vi "5.SFTP.vi"() -> ()   [LabVIEW 2012]
uses:
  UnderAutomation.UniversalRobots/UnderAutomation.UniversalRobots.lvlib
panel:
  in  "Directory to create":string
  out "Directory creation error":errorcluster
  in  "Create directory":bool
  out "Delete error":errorcluster
  in  "File or directory to delete":string
  in  "Delete":bool
  out "Download error":errorcluster
  out "Upload error":errorcluster
  out "List directory error":errorcluster
  in  "Upload":bool
  in  "Local Path":path
  in  "Robot Path":string
  in  "stop":bool
  in  "Robot Path":string
  out "DirectoryItems":T1(array[cluster])
  in  "List directory":bool
  in  "Download":bool
  out "Programs 2":string[](array[string])
  in  "Enumerate installations":bool
  in  "Enumerate programs":bool
  out "Programs":string[](array[string])
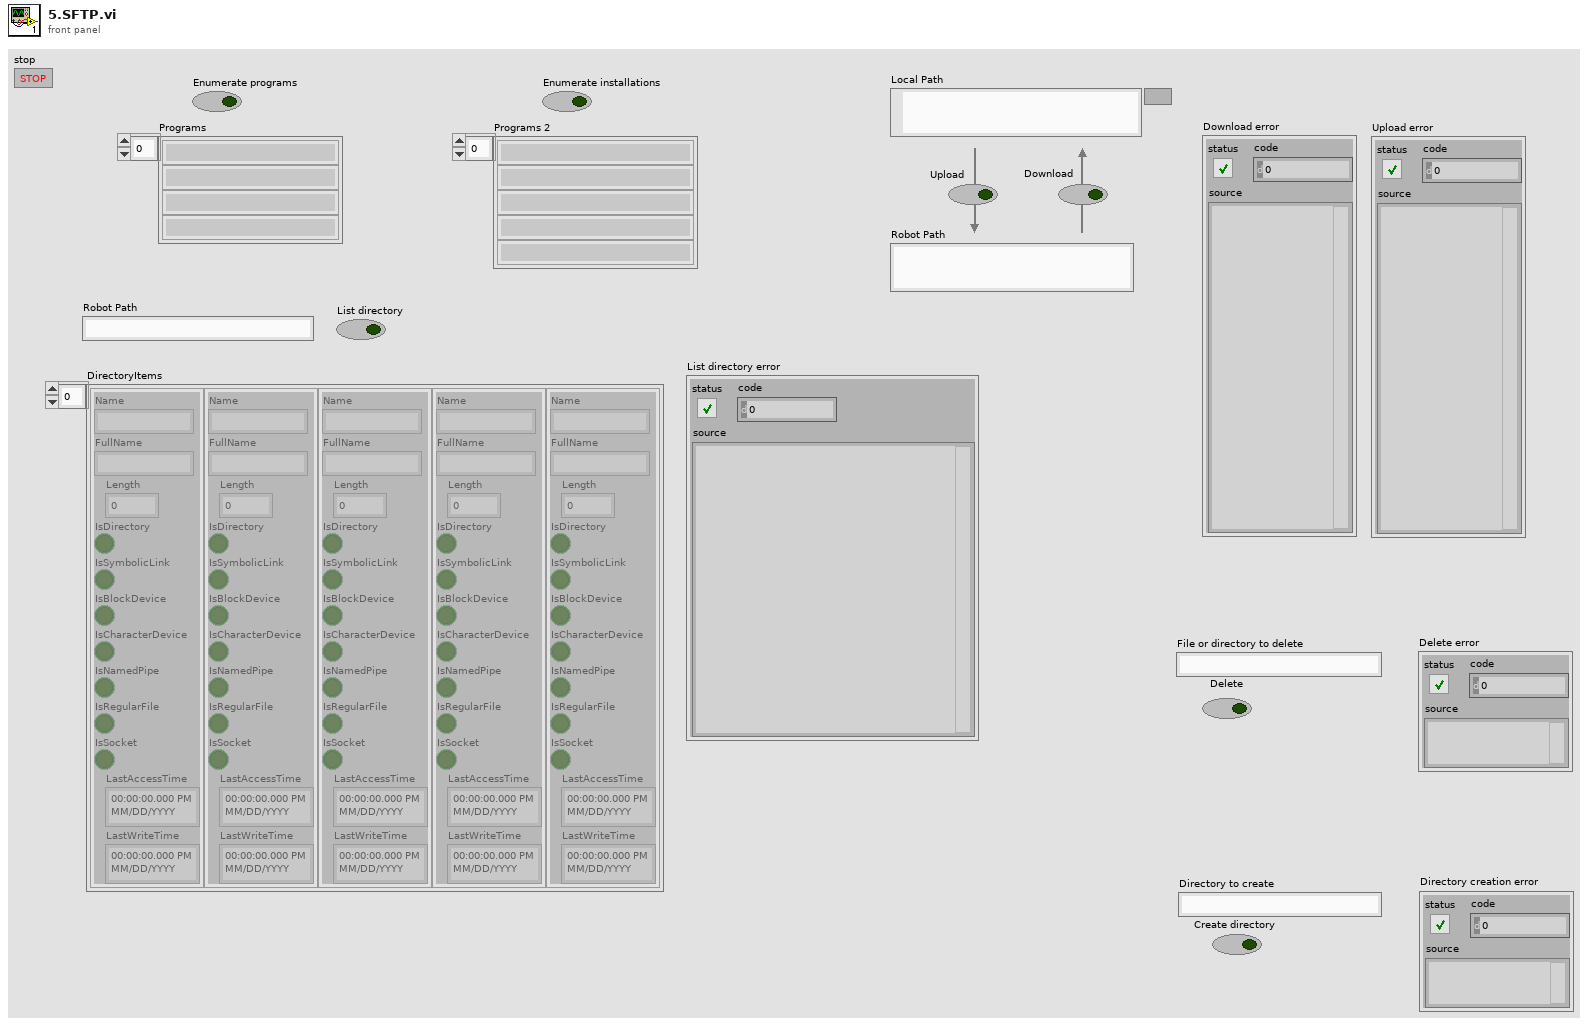
[diagram p1: front panel]
types:
  T1 = cluster{"Name":string, "FullName":string, "Length":i64, "IsDirectory":bool, "IsSymbolicLink":bool, "IsBlockDevice":bool, "IsCharacterDevice":bool, "IsNamedPipe":bool, "IsRegularFile":bool, "IsSocket":bool, "LastAccessTime":timestamp, "LastWriteTime":timestamp}[]
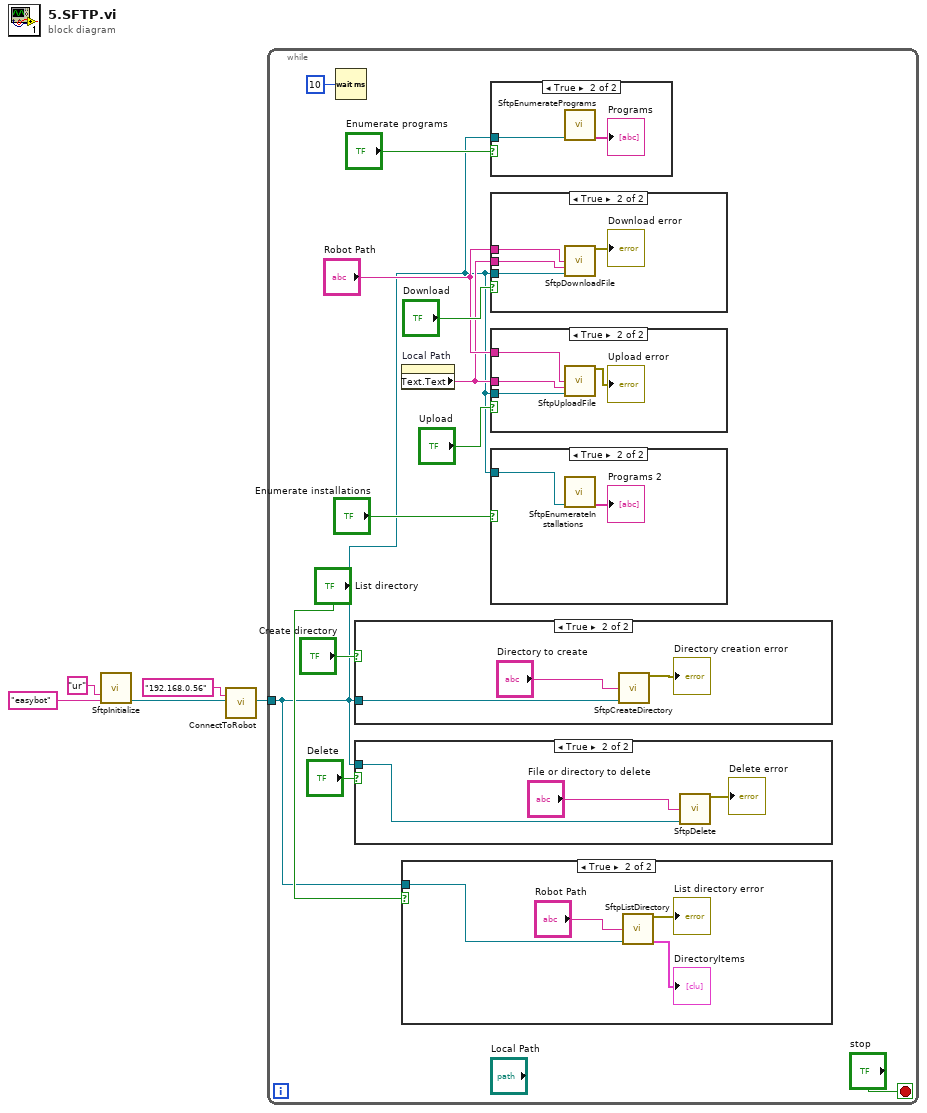
[diagram p0: block diagram]
diagram:
  n1 = call "SftpInitialize.vi"("Username"="ur", "Password"="easybot") -> ("SFTP Connect Parameters"=w3:refnum<k24>)  [unwired: 12 in, 1 out]
  n2 = call "ConnectToRobot.vi"("ip"="192.168.0.56", "SFTP Connect Parameters"=w3) -> ("Sftp"=w1:refnum<k24>)  [unwired: 12 in, 5 out]
  n3 = while {
    tunnel: w1 -> [w6]
    stop <- "stop" stop-if-true
    n4 = Wait (ms)(milliseconds to wait=u32 10) -> ()  [unwired: 1 out]
    n5 = case shown="True" "Create directory" {
      tunnel: w6 -> [_ w20]
      frame False {
      }
      frame True {
        n6 = call "SftpCreateDirectory.vi"("Robot Path"="Directory to create", "Sftp"=w20) -> ("error out"=→"Directory creation error":errorcluster)  [unwired: 13 in]
      }
    }
    n7 = case shown="True" "Delete" {
      tunnel: w6 -> [_ w21]
      frame False {
      }
      frame True {
        n8 = call "SftpDelete.vi"("Robot Path"="File or directory to delete", "Sftp"=w21) -> ("error out"=→"Delete error":errorcluster)  [unwired: 13 in]
      }
    }
    n9 = property on="Local Path" class="Path"() -> ("Text.Text"=w9:string)  [unwired: 2 in, 2 out]
    n10 = case shown="True" "List directory" {
      tunnel: w6 -> [_ w34]
      frame False {
      }
      frame True {
        n11 = call "SftpListDirectory.vi"("Robot Path"="Robot Path", "Sftp"=w34) -> ("error out"=→"List directory error":errorcluster, "DirectoryItems"=→"DirectoryItems":T1)  [unwired: 12 in]
      }
    }
    n12 = case shown="True" "Enumerate programs" {
      tunnel: w6 -> [_ w39]
      frame False {
      }
      frame True {
        n13 = call "SftpEnumeratePrograms.vi"("Sftp"=w39) -> ("Programs"=→"Programs":string[])  [unwired: 13 in, 1 out]
      }
    }
    n14 = case shown="True" "Download" {
      tunnel: w6 -> [_ w31]
      tunnel: "Robot Path" -> [_ w30]
      tunnel: w9 -> [_ w29]
      frame False {
      }
      frame True {
        n15 = call "SftpDownloadFile.vi"("Robot Path"=w30, "Local Path"=w29, "Sftp"=w31) -> ("error out"=→"Download error":errorcluster)  [unwired: 12 in]
      }
    }
    n16 = case shown="True" "Upload" {
      tunnel: "Robot Path" -> [_ w27]
      tunnel: w9 -> [_ w26]
      tunnel: w6 -> [_ w25]
      frame False {
      }
      frame True {
        n17 = call "SftpUploadFile.vi"("Robot Path"=w27, "Local Path"=w26, "Sftp"=w25) -> ("error out"=→"Upload error":errorcluster)  [unwired: 12 in]
      }
    }
    n18 = case shown="True" "Enumerate installations" {
      tunnel: w6 -> [_ w37]
      frame False {
      }
      frame True {
        n19 = call "SftpEnumerateInstallations.vi"("Sftp"=w37) -> ("Installations"=→"Programs 2":string[])  [unwired: 13 in, 1 out]
      }
    }
  }
